vi "Configure SA.vi"(0 "Refnum in":T1, 5 "Frequency Reference Source":string, 7 "External Attenuation":dbl, 9 "BLE  Channel":u8, 11 "error in (no error)":errorcluster) -> (4 "Refnum out":T1, 15 "error out":errorcluster)   [LabVIEW 2026, in "Nordic nRF52 DK DTM Test.lvlib"]
uses:
  Nordic nRF52 DK DTM Test.lvlib
  <vilib>/RFmx/RFInstr/mx/Support/RFmxInstrSupport.llb/niRFmx Instrument Handle.ctl
  <vilib>/RFmx/BT/mx/RFmxBT.llb/RFmxBT Configure IQ Power Edge Trigger.vi
  <resource>/objmgr/RFmxBT.rc
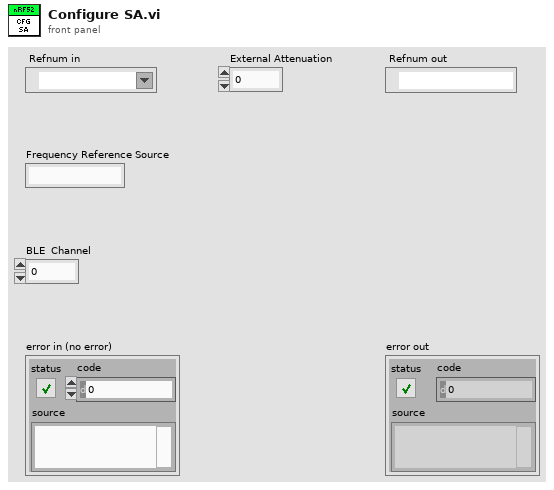
[diagram p1: front panel]
types:
  T1 = typedef "niRFmx Instrument Handle.ctl" = refnum<k21>
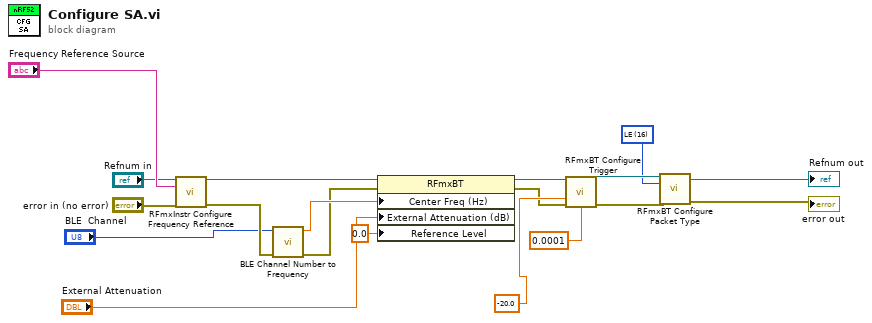
[diagram p0: block diagram]
diagram:
  w14 = 16 items=["DH1", "DH3", "DH5", "DM1", "DM3", "DM5", "2-DH1", "2-DH3", "2-DH5", "3-DH1", "3-DH3", "3-DH5", "2-EV3", "2-EV5", "3-EV3", "3-EV5", "LE", "LE-CS", "LE-HDT"] ("Packet Type")
  n1 = call <vilib>:"RFmxInstr Configure Frequency Reference.vi"("Instrument Handle In"="Refnum in", "Frequency Reference Source"="Frequency Reference Source", "error in (no error)"="error in (no error)") -> ("Instrument Handle Out"=w8:refnum<k21>, "error out"=w9:errorcluster)  [unwired: 11 in]
  n2 = call "BLE Channel Number to Frequency.vi"("error in (no error)"=w9, "BLE  Channel"="BLE  Channel") -> ("error out"=w10:errorcluster, "Frequency, Hz"=w11:dbl)  [unwired: 8 in]
  n3 = property class="RFmxBT"(reference=w8, error in=w10, "Center Freq (Hz)"=w11, "External Attenuation (dB)"="External Attenuation", "Reference Level"=0.0) -> (reference out=w15:refnum<k21>, error out=w3:errorcluster)
  n4 = call-poly <vilib>:"RFmxBT Configure Trigger.vi"("Instrument Handle In"=w15, "IQ Power Edge Level (dB or dBm)"=-20.0, "error in (no error)"=w3, "Minimum Quiet Time (s)"=0.0001) -> ("Instrument Handle Out"=w17:refnum<k21>, "error out"=w16:errorcluster)  [unwired: 10 in]
  n5 = call <vilib>:"RFmxBT Configure Packet Type.vi"("Instrument Handle In"=w17, "Packet Type"=w14, "error in (no error)"=w16) -> ("Instrument Handle Out"=→"Refnum out":refnum<k21>, "error out"=→"error out":errorcluster)  [unwired: 11 in]
